vi "Create RGB Color Scale Array.vi"() -> (2 "RGB Must Include":u32[](array[colorbox])=[16711680, 16776960, 65280, 65535, 255, 16711935], 3 "RGB Array":u32[](array[colorbox]))   [LabVIEW 2015, in "ColorSelector.lvclass"]
doc: "This VI creates the RGB Color Scale Array.\n<b> </b> <b> </b>\n©2017 Q Software Innovations, LLC (QSI)\nwritten by Quentin Alldredge\nproduced in LabVIEW 2015\n\nsupport@qsoftwareinnovations.com\nwww.qsoftwareinnovations.com\n\nAll rights reserved.\n\nRedistribution and use in source and binary forms, with or without modification, are permitted provided that the following conditions are met:\n\n * Redistributions of source code must retain the above copyright notice, this list of conditions and the following disclaimer.\n * Redistributions in binary form must reproduce the above copyright notice, this list of conditions and the following disclaimer in the documentation and/or other materials provided with the distribution.\n * Neither the name of Q Software Innovations, LLC. nor the names of its contributors may be used to endorse or promote products derived from this software without specific prior written permission.\n\nTHIS SOFTWARE IS PROVIDED BY THE COPYRIGHT HOLDERS AND CONTRIBUTORS \"AS IS\" AND ANY EXPRESS OR IMPLIED WARRANTIES, INCLUDING, BUT NOT LIMITED TO, THE IMPLIED WARRANTIES OF MERCHANTABILITY AND FITNESS FOR A PARTICULAR PURPOSE ARE DISCLAIMED. IN NO EVENT SHALL THE COPYRIGHT OWNER OR CONTRIBUTORS BE LIABLE FOR ANY DIRECT, INDIRECT, INCIDENTAL, SPECIAL, EXEMPLARY, OR CONSEQUENTIAL DAMAGES (INCLUDING, BUT NOT LIMITED TO, PROCUREMENT OF SUBSTITUTE GOODS OR SERVICES; LOSS OF USE, DATA, OR PROFITS; OR BUSINESS INTERRUPTION) HOWEVER CAUSED AND ON ANY THEORY OF LIABILITY, WHETHER IN CONTRACT, STRICT LIABILITY, OR TORT (INCLUDING NEGLIGENCE OR OTHERWISE) ARISING IN ANY WAY OUT OF THE USE OF THIS SOFTWARE, EVEN IF ADVISED OF THE POSSIBILITY OF SUCH DAMAGE."
uses:
  ColorSelector.lvclass
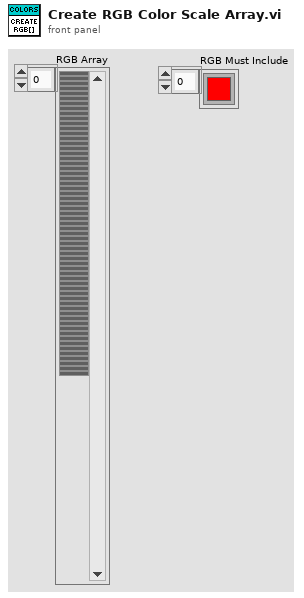
[diagram p1: front panel]
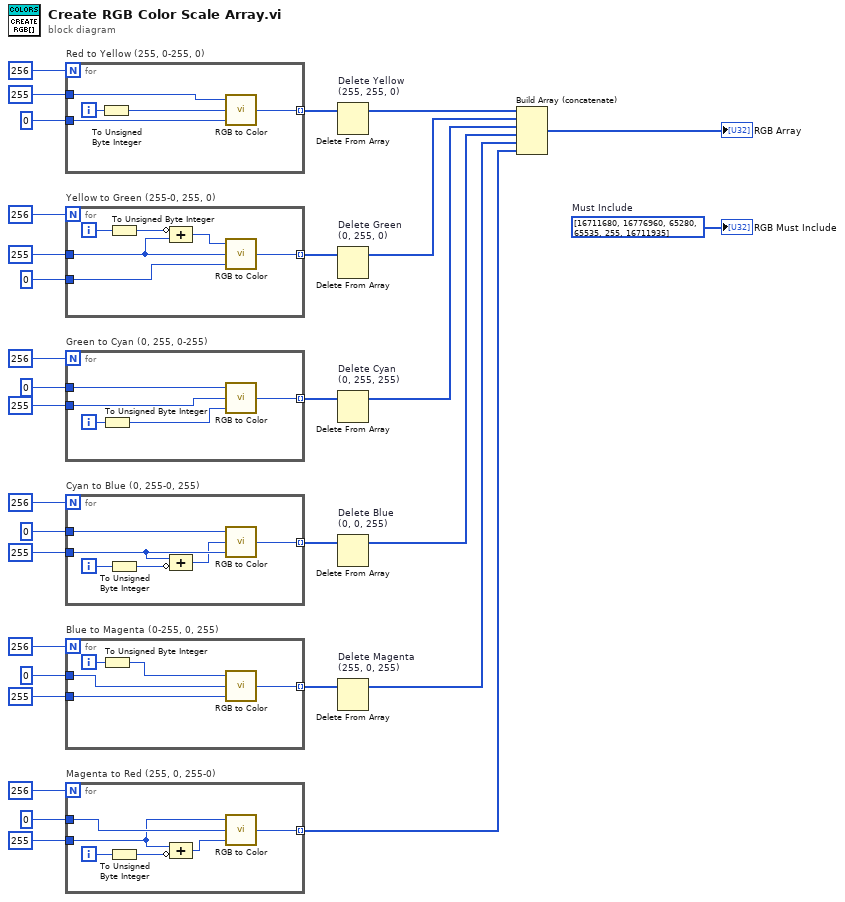
[diagram p0: block diagram]
diagram:
  w1 = u32[] [16711680, 16776960, 65280, 65535, 255, 16711935]  # Must Include
  n1 = for "Red to Yellow (255, 0-255, 0)" {
    N: 256 -> [_]
    tunnel: u8 255 -> [w35]
    tunnel: [w34] -> w30 mode=indexing
    tunnel: u8 0 ("B") -> [w33]
    i -> [w36]
    n2 = To Unsigned Byte Integer(number=w36) -> (unsigned 8bit integer=w32:u8)
    n3 = call <vilib>:"RGB to Color.vi"("B"=w33, "G"=w32, "R"=w35) -> ("Color"=w34:u32)
  }
  n4 = for "Yellow to Green (255-0, 255, 0)" {
    N: 256 -> [_]
    tunnel: u8 255 -> [w37]
    tunnel: [w42] -> w20 mode=indexing
    tunnel: u8 0 ("B") -> [w41]
    i -> [w39]
    n5 = To Unsigned Byte Integer(number=w39) -> (unsigned 8bit integer=w40:u8)
    n6 = Compound Arithmetic op=ADD(invert w40, w37) -> (w38:u8)
    n7 = call <vilib>:"RGB to Color.vi"("B"=w41, "G"=w37, "R"=w38) -> ("Color"=w42:u32)
  }
  n8 = for "Green to Cyan (0, 255, 0-255)" {
    N: 256 -> [_]
    tunnel: u8 255 -> [w46]
    tunnel: [w47] -> w15 mode=indexing
    tunnel: u8 0 ("B") -> [w45]
    i -> [w44]
    n9 = To Unsigned Byte Integer(number=w44) -> (unsigned 8bit integer=w43:u8)
    n10 = call <vilib>:"RGB to Color.vi"("B"=w43, "G"=w46, "R"=w45) -> ("Color"=w47:u32)
  }
  n11 = for "Cyan to Blue (0, 255-0, 255)" {
    N: 256 -> [_]
    tunnel: u8 255 -> [w49]
    tunnel: [w53] -> w10 mode=indexing
    tunnel: u8 0 ("B") -> [w52]
    i -> [w50]
    n12 = To Unsigned Byte Integer(number=w50) -> (unsigned 8bit integer=w51:u8)
    n13 = Compound Arithmetic op=ADD(w49, invert w51) -> (w48:u8)
    n14 = call <vilib>:"RGB to Color.vi"("B"=w49, "G"=w48, "R"=w52) -> ("Color"=w53:u32)
  }
  n15 = for "Blue to Magenta (0-255, 0, 255)" {
    N: 256 -> [_]
    tunnel: u8 255 -> [w56]
    tunnel: [w58] -> w5 mode=indexing
    tunnel: u8 0 ("B") -> [w55]
    i -> [w57]
    n16 = To Unsigned Byte Integer(number=w57) -> (unsigned 8bit integer=w54:u8)
    n17 = call <vilib>:"RGB to Color.vi"("B"=w56, "G"=w55, "R"=w54) -> ("Color"=w58:u32)
  }
  n18 = for "Magenta to Red (255, 0, 255-0)" {
    N: 256 -> [_]
    tunnel: u8 255 -> [w59]
    tunnel: [w64] -> w3 mode=indexing
    tunnel: u8 0 ("B") -> [w61]
    i -> [w62]
    n19 = To Unsigned Byte Integer(number=w62) -> (unsigned 8bit integer=w63:u8)
    n20 = Compound Arithmetic op=ADD(w59, invert w63) -> (w60:u8)
    n21 = call <vilib>:"RGB to Color.vi"("B"=w60, "G"=w61, "R"=w59) -> ("Color"=w64:u32)
  }
  n22 = Delete From Array "Delete Yellow \n(255, 255, 0)"(array=w30) -> (array with subset deleted=w24:u32[])  [unwired: 2 in, 1 out]
  n23 = Delete From Array "Delete Green \n(0, 255, 0)"(array=w20) -> (array with subset deleted=w19:u32[])  [unwired: 2 in, 1 out]
  n24 = Delete From Array "Delete Cyan \n(0, 255, 255)"(array=w15) -> (array with subset deleted=w14:u32[])  [unwired: 2 in, 1 out]
  n25 = Delete From Array "Delete Blue \n(0, 0, 255)"(array=w10) -> (array with subset deleted=w9:u32[])  [unwired: 2 in, 1 out]
  n26 = Delete From Array "Delete Magenta \n(255, 0, 255)"(array=w5) -> (array with subset deleted=w4:u32[])  [unwired: 2 in, 1 out]
  n27 = Build Array (concatenate)(w24, w19, w14, w9, w4, w3) -> (→"RGB Array":u32[])
  "RGB Must Include" <- w1
